vi "Manual Mode.vi"(8 "error in (no error)":errorcluster, 9 "Test Settings":T1, 10 "Model in":refnum<class "Model.lvclass">, 11 "Manual State in":refnum<class "Manual State.lvclass">) -> (0 "error out":errorcluster, 2 "Model out":refnum<class "Model.lvclass">, 3 "Manual State out":refnum<class "Manual State.lvclass">)   [LabVIEW 2016, in "Manual State.lvclass"]
uses:
  Manual State.lvclass
  Model/Model/Model.lvclass
  Typedefs/TestSettings.ctl
  Typedefs/HPMT_Typedefs.lvlib
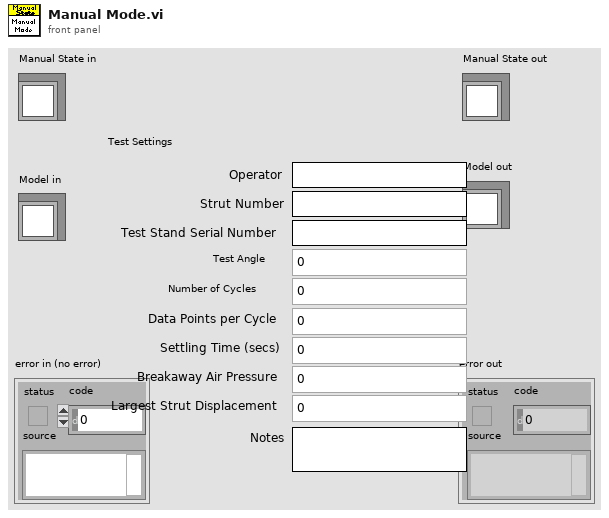
[diagram p1: front panel]
types:
  T1 = typedef "HPMT_Typedefs.lvlib/TestSettings.ctl" = cluster{"Operator":string, "Strut Number":string, "Test Stand Serial Number":string, "Notes":string, "Test Angle":u16, "Number of Cycles":u16, "Data Points per Cycle":u16, "Settling Time (secs)":u16, "Breakaway Air Pressure":u16, "Largest Strut Displacement":dbl}
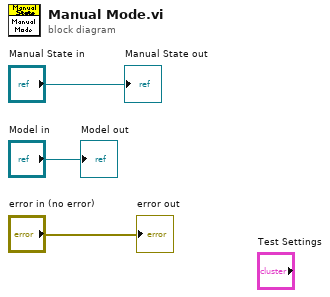
[diagram p0: block diagram]
diagram:
  "error out" <- "error in (no error)"
  "Manual State out" <- "Manual State in"
  "Model out" <- "Model in"
